vi "close.vi"(8 "error in (no error)":errorcluster, 11 "DmmKeysight in":refnum<class "DmmKeysight.lvclass">) -> (0 "error out":errorcluster)   [LabVIEW 2023, in "DmmKeysight.lvclass"]
doc: "<b>Author:</b> Wolfgang\n<b>Description:</b> This mimics the abilty to close an instrument reference if opened before."
uses:
  DmmKeysight.lvclass
  DmmKeysight.lvclass/DmmKeysight.ctl
  Multimeter.lvclass
  Driver/Keysight-34450A.lvlib
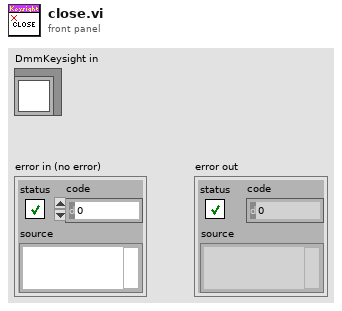
[diagram p1: front panel]
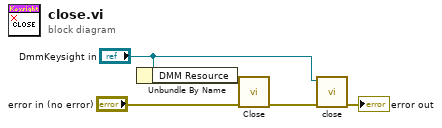
[diagram p0: block diagram]
diagram:
  n1 = Unbundle By Name("DmmKeysight in") -> ("DMM Resource"=w3:refnum<visa-resource-name>)
  n2 = call "Close.vi"("error in (no error)"="error in (no error)", "VISA resource name"=w3) -> ("error out"=w1:errorcluster)  [unwired: 9 in]
  n3 = call-parent "close.vi"("error in (no error)"=w1, "Instrument in"="DmmKeysight in") -> ("error out"=→"error out":errorcluster)  [unwired: 9 in]
